vi "Time taken bwtween part 1 and part 2 (AoC).vi"() -> ()   [LabVIEW 2021]
uses:
  64953d4e-c5d4-47e4-8c75-fb4e53b81e6b.vi
  <vilib>/regexp/Match Regular Expression.xnode
  <vilib>/Comparison/Less/Less Functor/Less Functor.lvclass
  <vilib>/Analysis/NI_AALBase.lvlib
panel:
  out "Time (Part1-Part2) - sorted":dbl[](graph)
  out "variance":dbl format="%0.2f"
  out "standard deviation":dbl format="%0.2f"
  out "mean":dbl format="%0.2f"
  out "Time (Part1-Part2)":dbl[](graph)
  out "Array":dbl[](array[numeric]) format="%#.1g"
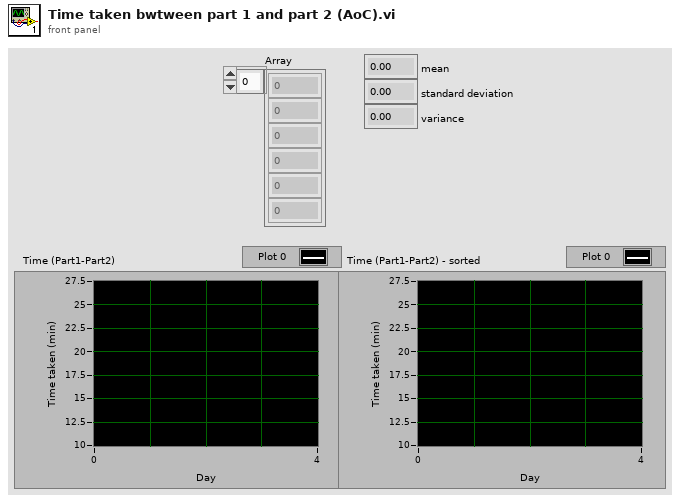
[diagram p1: front panel]
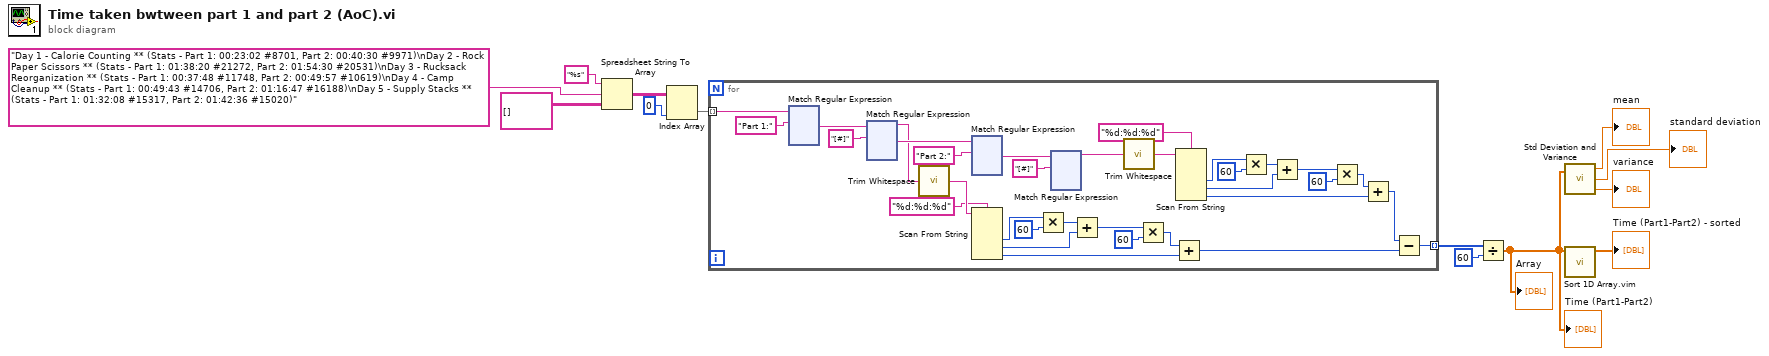
[diagram p0: block diagram]
diagram:
  n1 = Spreadsheet String To Array(format string="%s" ("delimiter (Tab)"), spreadsheet string="Day 1 - Calorie Counting ** (Stats - Part 1: 00:23:02 #8701, Part 2: 00:40:30 #9971)\nDay 2 - Rock Paper Scissors ** (Stats - Part 1: 01:38:20 #21272, Part 2: 01:54:30 #20531)\nDay 3 - Rucksack Reorganization ** (Stats - Part 1: 00:37:48 #11748, Part 2: 00:49:57 #10619)\nDay 4 - Camp Cleanup ** (Stats - Part 1: 00:49:43 #14706, Part 2: 01:16:47 #16188)\nDay 5 - Supply Stacks ** (Stats - Part 1: 01:32:08 #15317, Part 2: 01:42:36 #15020)" ("String"), array type (2D Dbl)=string[][] []) -> (array=w12:string[][])  [unwired: 1 in]
  n2 = Index Array(array=w12, index (col)=0 ("disabled index (col)")) -> (element=w9:string[])  [unwired: 1 in]
  n3 = for {
    tunnel: w9 -> [w15] mode=indexing
    tunnel: [w14] -> w7 mode=indexing
    n4 = xnode "Match Regular Expression"("input string"=w15, "regular expression"="Part 1:") -> ("after match"=w45:string)  [unwired: 4 in, 4 out]
    n5 = xnode "Match Regular Expression"("input string"=w45, "regular expression"="[#]") -> ("before match"=w38:string, "after match"=w41:string)  [unwired: 4 in, 3 out]
    n6 = call <vilib>:"Trim Whitespace.vi"("string"=w38) -> ("trimmed string"=w37:string)  [unwired: 1 in]
    n7 = xnode "Match Regular Expression"("input string"=w41, "regular expression"="Part 2:") -> ("after match"=w43:string)  [unwired: 4 in, 4 out]
    n8 = Scan From String(format string="%d:%d:%d", input string=w37) -> (output 1=w35:i32, output 2=w32:i32, output 3=w28:i32)  [unwired: 5 in, 3 out]
    n9 = Multiply(x=w35, y=60) -> (x*y=w33:i32)
    n10 = xnode "Match Regular Expression"("input string"=w43, "regular expression"="[#]") -> ("before match"=w40:string)  [unwired: 4 in, 4 out]
    n11 = Add(x=w33, y=w32) -> (x+y=w31:i32)
    n12 = call <vilib>:"Trim Whitespace.vi"("string"=w40) -> ("trimmed string"=w18:string)  [unwired: 1 in]
    n13 = Multiply(x=w31, y=60) -> (x*y=w29:i32)
    n14 = Add(x=w29, y=w28) -> (x+y=w16:i32)
    n15 = Scan From String(format string="%d:%d:%d", input string=w18) -> (output 1=w20:i32, output 2=w23:i32, output 3=w27:i32)  [unwired: 5 in, 3 out]
    n16 = Multiply(x=w20, y=60) -> (x*y=w22:i32)
    n17 = Add(x=w22, y=w23) -> (x+y=w24:i32)
    n18 = Multiply(x=w24, y=60) -> (x*y=w26:i32)
    n19 = Add(x=w26, y=w27) -> (x+y=w17:i32)
    n20 = Subtract(x=w17, y=w16) -> (x-y=w14:i32)
  }
  n21 = Divide(x=w7, y=60) -> (x/y=w2:dbl[])
  "Array" <- w2
  "Time (Part1-Part2)" <- w2
  n22 = call <vilib>:"Std Deviation and Variance.vi"("X"=w2) -> ("mean"=→"mean":dbl, "standard deviation"=→"standard deviation":dbl, "variance"=→"variance":dbl)  [unwired: 1 in]
  n23 = call "Sort 1D Array.vim"("unsorted array"=w2) -> ("sorted array"=→"Time (Part1-Part2) - sorted":dbl[])  [unwired: 10 in]
